vi "Return Stamp or Weight.vi"(8 "error in":errorcluster, 9 "Tool Type":enum16{"Stamp", "Weight"}(ring), 10 "Slot Number":i32, 11 "GrabberTool in":refnum<class "GrabberTool Class.lvclass">) -> (0 "error out":errorcluster, 3 "GrabberTool out":refnum<class "GrabberTool Class.lvclass">)   [LabVIEW 2011, in "GrabberTool Class.lvclass"]
uses:
  GrabberTool Class.lvclass
  Config Manager Class/Type Definitions/Named Position.ctl
  Config Manager Class/Type Definitions/Part Type.ctl
  Config Manager Class/Type Definitions/Offset.ctl
  WorkTable Class/WorkTable Class.lvclass
  Vec3d Class/Vec3d Class.lvclass
  Config Manager Class/Config Manager Class.lvclass
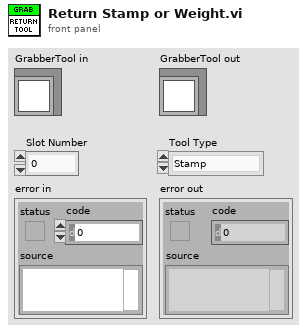
[diagram p1: front panel]
types:
  T1 = enum16{"Vertical First", "Lateral First", "Auto"}
  T2 = typedef "Named Position.ctl" = enum16{"home", "module_chuck_0", "module_chuck_1", "module_chuck_2", "module_chuck_3", "module_chuck_4", "glue_reservoir_chuck", "stamp_tool_chuck", "weight_tool_chuck", "needle_calibration", "tool_rack_pos_0_in", "tool_rack_pos_0_out", "tool_rack_pos_1_in", "tool_rack_pos_1_out", "tool_rack_pos_2_in", "tool_rack_pos_2_out", "front_load_position", "grabber_start_pos", "between_chuck_0_and_1", "between_chuck_2_and_3"}
  T3 = typedef "Part Type.ctl" = enum16{"BBM", "HDI", "BARE HDI", "GLUERESERVOIR", "STAMP_1", "STAMP_2", "STAMP_3", "STAMP_4", "STAMP_5", "WEIGHT_1", "WEIGHT_2", "WEIGHT_3", "WEIGHT_4", "WEIGHT_5", "WEIGHT_6", "WEIGHT_7", "WEIGHT_8", "PICKER_TOOL", "GRABER_TOOL"}
  T4 = typedef "Offset.ctl" = enum16{"needle_offset", "tool_holder_offset"}
  T5 = typedef "Worktable_Stamps.ctl" = cluster{"Stamp Slots":T6[], "Vacuum Channel":i32}
  T6 = typedef "Worktable_Stamp.ctl" = cluster{"Stamp State":enum16{"Empty", "Populated", "Used"}, "Location/Orientation":T7, "Stamp Type":T8}
  T7 = typedef "Position_Orientation.ctl" = cluster{"Center":refnum<class "Vec3d Class.lvclass">, "Orientation":refnum<class "Orient3d Class.lvclass">}
  T8 = typedef "Stamp Type.ctl" = enum16{"Stamp 1", "Stamp 2", "Stamp 3", "Stamp 4", "Stamp 5"}
  T9 = typedef "Worktable_Weights.ctl" = cluster{"Weight Slots":T10[], "Vacuum Channel":i32}
  T10 = typedef "Worktable_Weight.ctl" = cluster{"Weight State":enum16{"Empty", "Populated"}, "Weight Type":T11, "Location/Orientation":T7}
  T11 = typedef "Weight Type.ctl" = enum16{"Weight 1", "Weight 2", "Weight 3", "Weight 4", "Weight 5", "Weight 6", "Weight 7", "Weight 8"}
  T12 = typedef "Gluing Parameters.ctl" = cluster{"Safe Grabber Pickup":dbl, "Safe Grabber Lift":dbl, "Glue Resevoir Wait Time":dbl, "Glue BM Wait Time ":dbl, "Placed Weight X-Move":dbl}
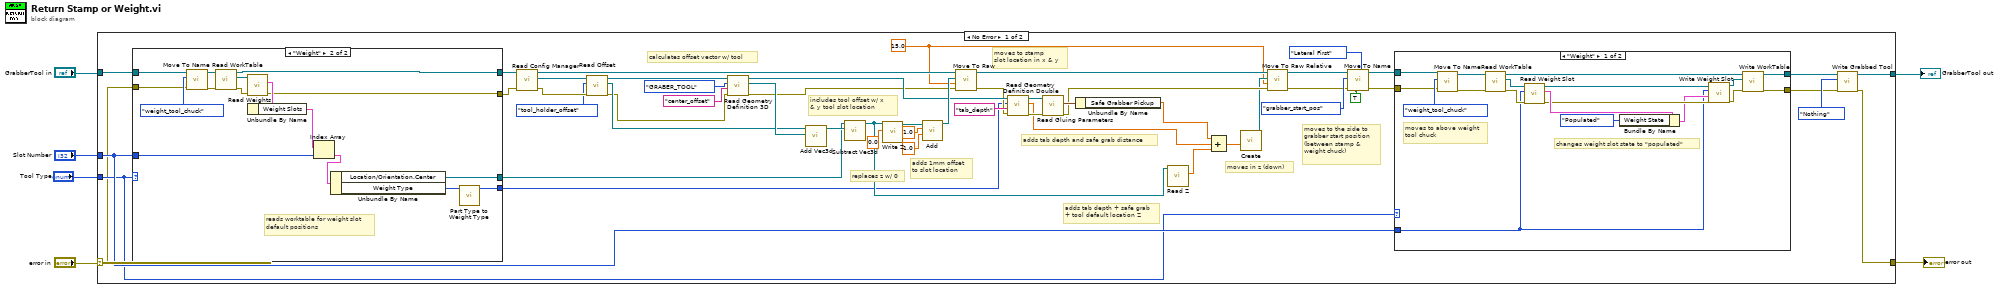
[diagram p0: block diagram]
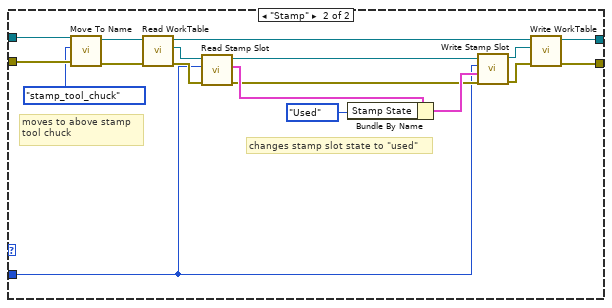
[diagram p2: hidden frame]
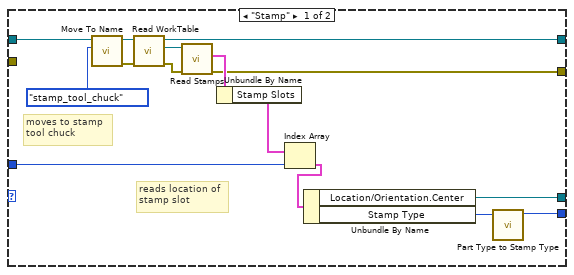
[diagram p3: hidden frame]
diagram:
  n1 = case shown="No Error" "error in" {
    selector: "error in" -> [w8 w127]
    tunnel: [w21 w127] -> w6
    tunnel: "GrabberTool in" -> [w15 w126]
    tunnel: "Slot Number" -> [w10 _]
    tunnel: [w22 w126] -> w4
    tunnel: "Tool Type" -> [w9 _]
    frame No Error {
      w17 = 15.0 ("Speed")
      # "moves to the side to\ngrabber start position\n(between stamp & \nweight chuck)"
      # "moves in z (down)"
      # "adds tab depth + safe grab\n+ tool default location Z"
      # "adds tab depth and safe grab distance"
      # "moves to stamp\nslot location in x & y"
      # "adds 1mm offset\nto slot location"
      # "includes tool offset w/ x \n& y tool slot location"
      # "replaces z w/ 0"
      # "calculates offset vector w/ tool"
      n2 = case shown="\"Weight\"" w9 {
        tunnel: w15 -> [w101 w125]
        tunnel: [w100 w120] -> w14
        tunnel: [w99 w114] -> w13
        tunnel: w10 -> [w98 w117]
        tunnel: [w96 w113] -> w12
        tunnel: [w95 w111] -> w11
        tunnel: w8 -> [_ w110]
        frame "Stamp" {
          # "reads location of\nstamp slot"
          # "moves to stamp\ntool chuck"
          n3 = call-dynamic "Move To Name.vi"("Destination"=Named_Position."stamp_tool_chuck", "Gantry in"=w101) -> ("error out"=w104:errorcluster, "Gantry out"=w103:refnum<class "GrabberTool Class.lvclass">)  [unwired: 8 in]
          n4 = call-dynamic "Read WorkTable.vi"("error in"=w104, "Gantry Class in"=w103) -> ("error out"=w106:errorcluster, "WorkTable Class.lvclass"=w105:refnum<class "WorkTable Class.lvclass">, "Gantry Class out"=w100:refnum<class "GrabberTool Class.lvclass">)  [unwired: 7 in]
          n5 = call-dynamic "Read Stamps.vi"("error in (no error)"=w106, "WorkTable Class in"=w105) -> ("error out"=w99:errorcluster, "Stamps"=w107:T5)  [unwired: 7 in, 1 out]
          n6 = Unbundle By Name(w107) -> ("Stamp Slots"=w108:T6[])
          n7 = Index Array(array=w108, index=w98) -> (element=w109:T6)
          n8 = Unbundle By Name(w109) -> ("Location/Orientation.Center"=w96:refnum<class "Vec3d Class.lvclass">, "Stamp Type"=w97:T8)
          n9 = call "Part Type to Stamp Type.vi"("Stamp Type"=w97) -> ("Part Type"=w95:T3)  [unwired: 9 in, 1 out]
        }
        frame "Weight" {
          # "reads worktable for weight slot\ndefault positions"
          n10 = call-dynamic "Move To Name.vi"("error in"=w110, "Destination"=Named_Position."weight_tool_chuck", "Gantry in"=w125) -> ("error out"=w122:errorcluster, "Gantry out"=w123:refnum<class "GrabberTool Class.lvclass">)  [unwired: 7 in]
          n11 = call-dynamic "Read WorkTable.vi"("error in"=w122, "Gantry Class in"=w123) -> ("error out"=w115:errorcluster, "WorkTable Class.lvclass"=w121:refnum<class "WorkTable Class.lvclass">, "Gantry Class out"=w120:refnum<class "GrabberTool Class.lvclass">)  [unwired: 7 in]
          n12 = call-dynamic "Read Weights.vi"("error in (no error)"=w115, "WorkTable Class in"=w121) -> ("error out"=w114:errorcluster, "Weights"=w119:T9)  [unwired: 7 in, 1 out]
          n13 = Unbundle By Name(w119) -> ("Weight Slots"=w118:T10[])
          n14 = Index Array(array=w118, index=w117) -> (element=w116:T10)
          n15 = Unbundle By Name(w116) -> ("Location/Orientation.Center"=w113:refnum<class "Vec3d Class.lvclass">, "Weight Type"=w112:T11)
          n16 = call "Part Type to Weight Type.vi"("Weight Type"=w112) -> ("Part Type"=w111:T3)  [unwired: 9 in, 1 out]
        }
      }
      n17 = call-dynamic "Read Config Manager.vi"("error in"=w13, "Gantry in"=w14) -> ("error out"=w57:errorcluster, "Config Manager"=w58:refnum<class "Config Manager Class.lvclass">, "Gantry out"=w49:refnum<class "GrabberTool Class.lvclass">)  [unwired: 7 in]
      n18 = call "Read Offset.vi"("error in"=w57, "Offset"=Offset."tool_holder_offset", "Config Manager in"=w58) -> ("error out"=w16:errorcluster, "Vec3d out"=w51:refnum<class "Vec3d Class.lvclass">, "Config Manager out"=w55:refnum<class "Config Manager Class.lvclass">)  [unwired: 6 in]
      n19 = call "Read Geometry Definition 3D.vi"("error in"=w16, "Feature"="center_offset", "Part Type"=Part_Type."GRABER_TOOL", "Config Manager in"=w55) -> ("error out"=w42:errorcluster, "Feature Coordinates"=w52:refnum<class "Vec3d Class.lvclass">, "Config Manager out"=w45:refnum<class "Config Manager Class.lvclass">)  [unwired: 5 in]
      n20 = call-dynamic "Add Vec3d.vi"(10:"Vec3d Class in"=w52, 11:"Vec3d Class in"=w51) -> ("Vec3d Class out"=w29:refnum<class "Vec3d Class.lvclass">)  [unwired: 8 in, 1 out]
      n21 = call "Subtract Vec3d.vi"("Vec3d in 2"=w29, "Vec3d in 1"=w12) -> ("Vec3d Class out"=w20:refnum<class "Vec3d Class.lvclass">)  [unwired: 8 in, 1 out]
      n22 = call-dynamic "Write Z.vi"("Z"=0.0, "Vec3d Class in"=w20) -> ("Vec3d Class out"=w30:refnum<class "Vec3d Class.lvclass">)  [unwired: 8 in, 1 out]
      n23 = call-dynamic "Add.vi"("Y"=1.0, "X"=1.0, "Vec3d in"=w30) -> ("Vec3d out"=w48:refnum<class "Vec3d Class.lvclass">)  [unwired: 6 in, 1 out]
      n24 = call-dynamic "Move To Raw.vi"("error in"=w42, "Speed"=w17, "Destination"=w48, "Gantry in"=w49) -> ("error out"=w41:errorcluster, "Gantry out"=w38:refnum<class "GrabberTool Class.lvclass">)  [unwired: 6 in]
      n25 = call "Read Geometry Definition Double.vi"("error in"=w41, "Feature"="tab_depth", "Part Type"=w11, "Config Manager in"=w45) -> ("error out"=w40:errorcluster, "Geometry Definition"=w27:dbl, "Config Manager out"=w44:refnum<class "Config Manager Class.lvclass">)  [unwired: 5 in]
      n26 = call "Read Gluing Parameters.vi"("error in (no error)"=w40, "Config Manager Class in"=w44) -> ("error out"=w37:errorcluster, "Gluing Parameters"=w39:T12)  [unwired: 7 in, 1 out]
      n27 = Unbundle By Name(w39) -> ("Safe Grabber Pickup"=w28:dbl)
      n28 = call-dynamic "Read Z.vi"("Vec3d Class in"=w20) -> ("Z"=w26:dbl)  [unwired: 8 in, 2 out]
      n29 = Compound Arithmetic op=ADD(w28, w27, w26) -> (w25:dbl)
      n30 = call "Create.vi"("Z"=w25) -> ("Vec3d Class out"=w36:refnum<class "Vec3d Class.lvclass">)  [unwired: 9 in, 1 out]
      n31 = call-dynamic "Move To Raw Relative.vi"("error in"=w37, "Speed(mm/s)"=w17, "Delta"=w36, "Gantry in"=w38) -> ("error out"=w33:errorcluster, "Gantry out"=w35:refnum<class "GrabberTool Class.lvclass">)  [unwired: 6 in]
      n32 = call-dynamic "Move To Name.vi"("Motion Order"=T1."Lateral First", "Direct"=TRUE, "error in"=w33, "Destination"=Named_Position."grabber_start_pos", "Gantry in"=w35) -> ("error out"=w31:errorcluster, "Gantry out"=w32:refnum<class "GrabberTool Class.lvclass">)  [unwired: 5 in]
      n33 = case shown="\"Weight\"" w9 {
        tunnel: w32 -> [w65 w94]
        tunnel: w31 -> [w64 w93]
        tunnel: [w61 w79] -> w19
        tunnel: [w60 w78] -> w18
        tunnel: w10 -> [w59 w77]
        frame "Weight" {
          # "changes weight slot state to \"populated\""
          # "moves to above weight\ntool chuck"
          n34 = call-dynamic "Move To Name.vi"("error in"=w64, "Destination"=Named_Position."weight_tool_chuck", "Gantry in"=w65) -> ("error out"=w74:errorcluster, "Gantry out"=w75:refnum<class "GrabberTool Class.lvclass">)  [unwired: 7 in]
          n35 = call-dynamic "Read WorkTable.vi"("error in"=w74, "Gantry Class in"=w75) -> ("error out"=w69:errorcluster, "WorkTable Class.lvclass"=w72:refnum<class "WorkTable Class.lvclass">, "Gantry Class out"=w73:refnum<class "GrabberTool Class.lvclass">)  [unwired: 7 in]
          n36 = call "Read Weight Slot.vi"("error in (no error)"=w69, "weight slot"=w59, "WorkTable Class in"=w72) -> ("error out"=w68:errorcluster, "Weight Slot"=w71:T10, "WorkTable Class out"=w70:refnum<class "WorkTable Class.lvclass">)  [unwired: 6 in]
          n37 = Bundle By Name(cluster=w71, "Weight State"=enum16{"Empty", "Populated"}."Populated") -> (w62:T10)
          n38 = call "Write Weight Slot.vi"("error in (no error)"=w68, "Weight Slot"=w62, "weight slot"=w59, "WorkTable Class in"=w70) -> ("error out"=w67:errorcluster, "WorkTable Class out"=w66:refnum<class "WorkTable Class.lvclass">)  [unwired: 6 in]
          n39 = call-dynamic "Write WorkTable.vi"("error in (no error)"=w67, "WorkTable Class.lvclass"=w66, "Gantry Class in"=w73) -> ("error out"=w60:errorcluster, "Gantry Class out"=w61:refnum<class "GrabberTool Class.lvclass">)  [unwired: 7 in]
        }
        frame "Stamp" {
          # "changes stamp slot state to \"used\""
          # "moves to above stamp\ntool chuck"
          n40 = call-dynamic "Move To Name.vi"("error in"=w93, "Destination"=Named_Position."stamp_tool_chuck", "Gantry in"=w94) -> ("error out"=w90:errorcluster, "Gantry out"=w91:refnum<class "GrabberTool Class.lvclass">)  [unwired: 7 in]
          n41 = call-dynamic "Read WorkTable.vi"("error in"=w90, "Gantry Class in"=w91) -> ("error out"=w84:errorcluster, "WorkTable Class.lvclass"=w88:refnum<class "WorkTable Class.lvclass">, "Gantry Class out"=w89:refnum<class "GrabberTool Class.lvclass">)  [unwired: 7 in]
          n42 = call "Read Stamp Slot.vi"("error in (no error)"=w84, "Stamp Slot"=w77, "WorkTable Class in"=w88) -> ("error out"=w83:errorcluster, "Stamp Slot"=w87:T6, "WorkTable Class out"=w86:refnum<class "WorkTable Class.lvclass">)  [unwired: 6 in]
          n43 = Bundle By Name(cluster=w87, "Stamp State"=enum16{"Empty", "Populated", "Used"}."Used") -> (w85:T6)
          n44 = call "Write Stamp Slot.vi"("error in (no error)"=w83, 9:"Stamp Slot"=w85, 10:"Stamp Slot"=w77, "WorkTable Class in"=w86) -> ("error out"=w82:errorcluster, "WorkTable Class out"=w81:refnum<class "WorkTable Class.lvclass">)  [unwired: 6 in]
          n45 = call-dynamic "Write WorkTable.vi"("error in (no error)"=w82, "WorkTable Class.lvclass"=w81, "Gantry Class in"=w89) -> ("error out"=w78:errorcluster, "Gantry Class out"=w79:refnum<class "GrabberTool Class.lvclass">)  [unwired: 7 in]
        }
      }
      n46 = call "Write Grabbed Tool.vi"("error in (no error)"=w18, "Grabbed Tool"=enum16{"Weight Tool", "Stamp Tool", "Nothing"}."Nothing", "GrabberTool Class in"=w19) -> ("error out"=w21:errorcluster, "GrabberTool Class out"=w22:refnum<class "GrabberTool Class.lvclass">)  [unwired: 7 in]
    }
    frame Error {
    }
  }
  "error out" <- w6
  "GrabberTool out" <- w4
